vi "Real Time Clock - DS1307.vi"() -> ()   [LabVIEW 2011, in "LVH-LINX.lvlib"]
uses:
  vi.lib/LabVIEW Hacker/LINX/LVH-LINX.lvlib
  vi.lib/LabVIEW Hacker/LINX/Public/Sensors/DS1307/DS1307.lvlib
panel:
  out "Loop Rate (Hz)":u32
  in  "Serial Port":refnum<visa-resource-name>
  in  "Stop Button":bool
  out "DS1307 Time Stamp":timestamp
  # "LINX Device Settings"
  # "DS1307 Time Stamp"
  # "DS1307 Real-Time Clock Example (Serial Interface)\n\nThis example demonstrates how to set DS1307's time to the current system time.  \nThe time is then read back from the DS1307 and displayed on the front panel.\n\nInstructions\n1. Select the COM Port associated with the LINX Device.\n2. Click the Run Arrow."
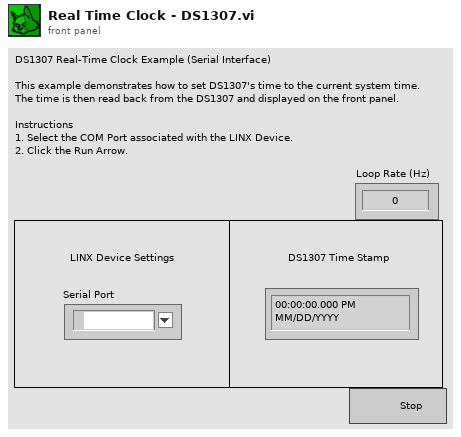
[diagram p1: front panel]
types:
  T1 = typedef "LVH-LINX.lvlib/LINX Ref.ctl" = cluster{"Platform":T2, "Interface":T3, "LINX Device Config":T4}
  T2 = typedef "LVH-LINX.lvlib/Platform.ctl" = enum16{"LINX", "myRIO"}
  T3 = typedef "LVH-LINX.lvlib/Interface.ctl" = enum16{"Serial", "TCP"}
  T4 = typedef "LVH-LINX.lvlib/Device.lvlib/LINX Device Config.ctl" = cluster{"Interface":T3, "COM Port":refnum<visa-resource-name>, "TCP Configuration":T5, "Device Family":T6, "Device ID":u8, "Device Name":string, "TCP Ref":refnum<k5>}
  T5 = typedef "LVH-LINX.lvlib/Device.lvlib/TCP Config.ctl" = cluster{"IP Address":string, "Port":u16}
  T6 = typedef "LVH-LINX.lvlib/Device Family.ctl" = enum8{"National Instruments", "Digilent", "Arduino"}
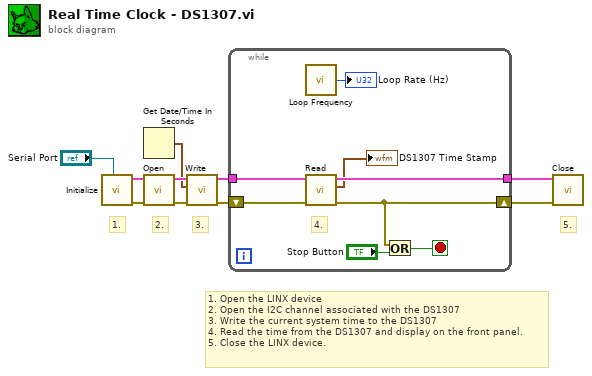
[diagram p0: block diagram]
diagram:
  # "5."
  # "3."
  # "2."
  # "1."
  # "1. Open the LINX device\n2. Open the I2C channel associated with the DS1307\n3. Write the current system time to the DS1307\n4. Read the time from the DS1307 and display on the front panel.\n5. Close the LINX device."
  n1 = call "Initialize.vi"("Serial Port"="Serial Port") -> ("Error Out"=w10:errorcluster, "LINX Ref"=w7:T1)  [unwired: 8 in, 1 out]
  n2 = Get Date/Time In Seconds() -> (seconds since 1Jan1904=w6:timestamp)
  n3 = call "Open.vi"("Error In"=w10, "LINX Resource"=w7) -> ("Error Out"=w9:errorcluster, "LINX Resource"=w8:T1)  [unwired: 8 in]
  n4 = call "Write.vi"("Error In"=w9, "Time Stamp"=w6, "LINX Resource"=w8) -> ("Error Out"=w4:errorcluster, "LINX Resource"=w5:T1)  [unwired: 7 in]
  n5 = while {
    tunnel: w5 -> [w18]
    tunnel: [w16] -> w2
    shift-right: [w12] -> w3
    shift-left: w4 -> [w17]
    stop <- w14 stop-if-true
    # "4."
    n6 = call "Loop Frequency.vi"() -> ("Loop Rate (Hz)"=→"Loop Rate (Hz)":u32)
    n7 = call "Read.vi"("Error In"=w17, "LINX Resource"=w18) -> ("Error Out"=w12:errorcluster, "Time Stamp"=→"DS1307 Time Stamp":timestamp, "LINX Resource"=w16:T1)  [unwired: 7 in]
    n8 = Or(x=w12, y="Stop Button") -> (x .or. y?=w14:bool)
  }
  n9 = call "Close.vi"("Error In"=w3, "LINX Resource"=w2) -> ()  [unwired: 8 in, 2 out]
